vi "extractObjectPrivateDataValues.vi"(7 "error in (no error)":errorcluster, 8 "classPrivateDataDefaults":variant[](array[variant]), 9 "Object in":refnum<class>) -> (0 "error out":errorcluster, 2 "objectPrivateData":variant[](array[variant]))   [LabVIEW 2020, in "JKI JSON Object Serialization.lvlib" / "OOP_Utility.lvlib" / "Reflection.lvclass"]
doc: "Returns object Private Data values for the complete class hierarchy.\nClass Private Data defaults must be passed as an array of Variants where each element is a cluster of class private data with element 0 being the current class and the last element is the top ancestor class.\n\nGCraftsman JSON Object Serialization Toolkit\nwww.GCraftsman.com\nCopyright (c) 2017, GCraftsman"
uses:
  Reflection.lvclass
  Reflection.lvclass/Reflection.ctl
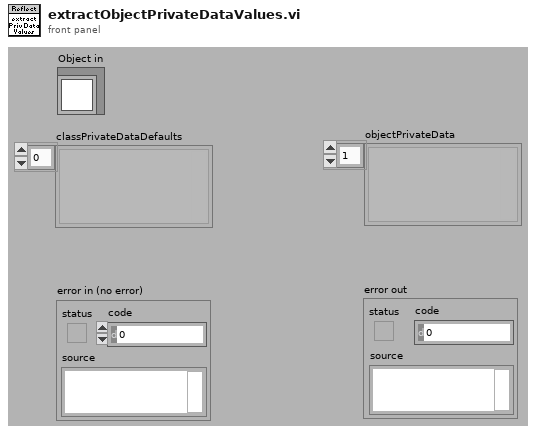
[diagram p1: front panel]
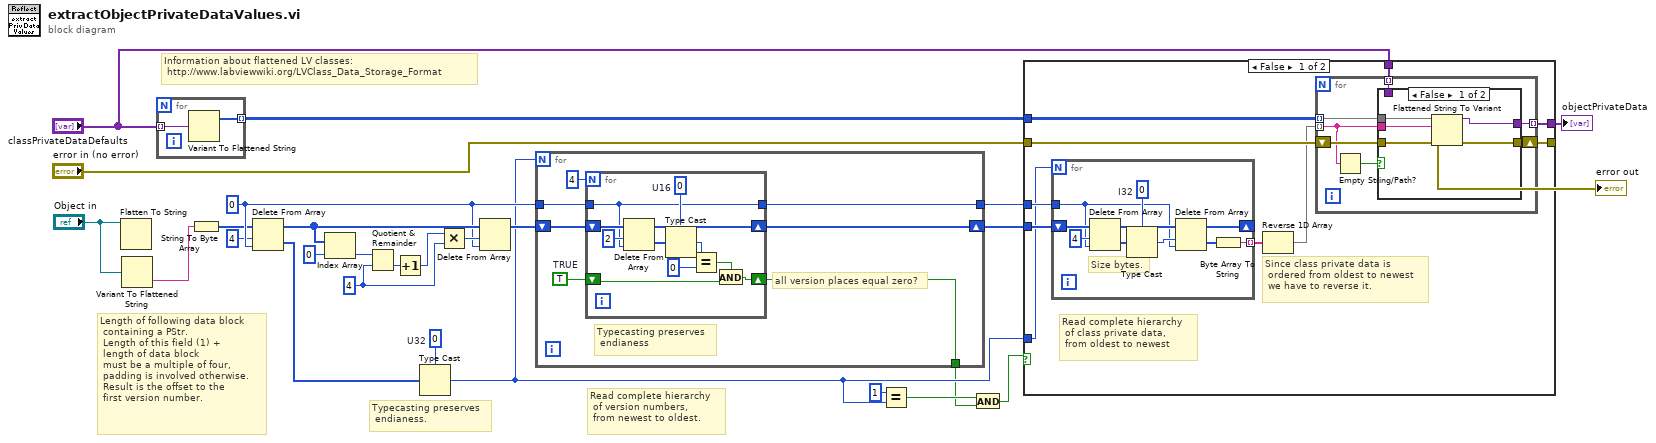
[diagram p0: block diagram]
diagram:
  w5 = u32 0  # U32
  w9 = u8 4 ("y")
  w20 = 0 ("index")
  # "Read complete hierarchy\n of version numbers,\n from newest to oldest."
  # "Information about flattened LV classes:\n http://www.labviewwiki.org/LVClass_Data_Storage_Format"
  # "Typecasting preserves\n endianess."
  # "Length of following data block\n containing a PStr.\n Length of this field (1) +\n length of data block\n must be a multiple of four,\n padding is involved otherwise.\n Result is the offset to the\n first version number."
  n1 = Flatten To String(anything="Object in") -> ()  [unwired: 3 in, 3 out]
  n2 = Variant To Flattened String(Variant="Object in") -> (data string=w1:string)  [unwired: 1 out]
  n3 = for {
    tunnel: [w29] -> w15 mode=indexing
    tunnel: "classPrivateDataDefaults" -> [w28] mode=indexing
    n4 = Variant To Flattened String(Variant=w28) -> (1:w29:i16[])  [unwired: 1 out]
  }
  n5 = String To Byte Array(string=w1) -> (unsigned byte array=w17:u8[])
  n6 = Delete From Array(array=w17, length=4 ("offset (0)"), index=w20) -> (deleted portion=w7:u8[], array with subset deleted=w23:u8[])
  n7 = Index Array(array=w23, index=0) -> (element=w12:u8)
  n8 = Quotient & Remainder(x=w12, y=w9) -> (floor(x/y)=w11:u8)  [unwired: 1 out]
  n9 = Increment(x=w11) -> (x+1=w10:u8)
  n10 = Type Cast(type=w5, x=w7) -> (*(type *) &x=w6:u32)
  n11 = Multiply(x=w10, y=w9) -> (x*y=w22:u8)
  n12 = Delete From Array(array=w23, length=w22, index=w20) -> (array with subset deleted=w18:u8[])  [unwired: 1 out]
  n13 = for {
    N: w6 -> [_]
    shift-right: [w35] -> w19
    shift-left: w18 -> [w36]
    tunnel: w20 -> [w34]
    tunnel: [w33] -> w21
    tunnel: [w30] -> w3
    w31 = TRUE  # TRUE
    # "all version places equal zero?"
    # "Typecasting preserves\n endianess"
    n14 = for {
      N: 4 -> [_]
      shift-right: [w45] -> w35
      shift-left: w36 -> [w47]
      tunnel: w34 -> [w42]
      tunnel: [w42] -> w33
      shift-right: [w37] -> w30
      shift-left: w31 -> [w38]
      w43 = u16 0  # U16
      n15 = Delete From Array(array=w47, length=2, index=w42) -> (deleted portion=w44:u8[], array with subset deleted=w45:u8[])
      n16 = Type Cast(type=w43, x=w44) -> (*(type *) &x=w41:u16)
      n17 = Equal?(x=w41, y=u16 0) -> (x = y?=w39:bool)
      n18 = And(x=w39, y=w38) -> (x .and. y?=w37:bool)
    }
  }
  n19 = Equal?(x=u32 1, y=w6) -> (x = y?=w25:bool)
  n20 = And(x=w25, y=w3) -> (x .and. y?=w26:bool)
  n21 = case shown="False" w26 {
    tunnel: w15 -> [w57 _]
    tunnel: [w52 w83] -> w27
    tunnel: w19 -> [w56 _]
    tunnel: w21 -> [w55 _]
    tunnel: w6 -> [w54 _]
    tunnel: [w53 w82] -> w14
    tunnel: "error in (no error)" -> [w51 w82]
    tunnel: "classPrivateDataDefaults" -> [w48 w83]
    frame False {
      # "Since class private data is\n ordered from oldest to newest\n we have to reverse it."
      # "Read complete hierarchy\n of class private data,\n from oldest to newest"
      n22 = for {
        N: w54 -> [_]
        shift-right: [w76] -> _
        shift-left: w56 -> [w81]
        tunnel: w55 -> [w74]
        tunnel: [w72] -> w50 mode=indexing
        w79 = 0  # I32
        # "Size bytes."
        n23 = Delete From Array(array=w81, length=4, index=w74) -> (deleted portion=w78:u8[], array with subset deleted=w77:u8[])
        n24 = Type Cast(type=w79, x=w78) -> (*(type *) &x=w75:i32)
        n25 = Delete From Array(array=w77, length=w75, index=w74) -> (deleted portion=w73:u8[], array with subset deleted=w76:u8[])
        n26 = Byte Array To String(unsigned byte array=w73) -> (string=w72:string)
      }
      n27 = Reverse 1D Array(array=w50) -> (reversed array=w49:string[])
      n28 = for {
        tunnel: w57 -> [w64] mode=indexing
        tunnel: [w61] -> w52 mode=indexing
        tunnel: w49 -> [w60] mode=indexing
        shift-right: [w62] -> w53
        shift-left: w51 -> [w63]
        tunnel: w48 -> [w58] mode=indexing
        n29 = Empty String/Path?(string/path=w60) -> (empty?=w59:bool)
        n30 = case shown="False" w59 {
          tunnel: w64 -> [w69 _]
          tunnel: w63 -> [w68 w70]
          tunnel: w60 -> [w67 _]
          tunnel: [w66 w70] -> w62
          tunnel: [w65 w71] -> w61
          tunnel: w58 -> [_ w71]
          frame False {
            n31 = Flattened String To Variant(4:w68, 6:w67, 7:w69) -> (0:w66:errorcluster, 3:w65:variant)
          }
          frame True {
            # "No data in this object.\nUse default value."
          }
        }
      }
    }
    frame True {
      # "// Version equals 0.0.0.0 and inheritance level is 1 (parent is LV object).\n// This means the private data cluster of the input object is empty.\n// Thus we return the default class private data"
    }
  }
  "objectPrivateData" <- w27
  "error out" <- w14
